vi "aal_Complex Modulator with Phase (complex input).vi"(7 "reset ?":bool, 8 "initial phase":dbl, 9 "fs":dbl=1024.0 min=-0.5 max=0.5 format="%.2f", 10 "frequency":dbl min=-0.5 max=0.5 format="%.2f", 11 "x":cdb[](array[numeric])) -> (3 "y":cdb[](array[numeric]))   [LabVIEW 2020, in "NI_AAL_SigProc.lvlib"]
doc: "Modulates the signal to frequency. The center frequency should be normalized (-0.5, 0.5)."
uses:
  <vilib>/Analysis/NI_AAL_SigProc.lvlib
  <resource>/lvanlys.dll
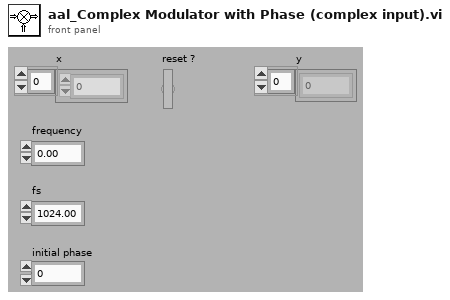
[diagram p1: front panel]
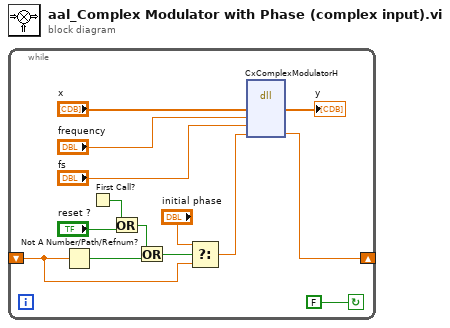
[diagram p0: block diagram]
diagram:
  n1 = while {
    shift-left: _ -> [w14]
    shift-right: [w9] -> _
    stop <- FALSE continue-if-true
    n2 = Not A Number/Path/Refnum?(number/path/refnum=w14) -> (NaN/Path/Refnum?=w5:bool)
    n3 = First Call?() -> (First Call?: T/F=w3:bool)
    n4 = Or(x=w3, y="reset ?") -> (x .or. y?=w1:bool)
    n5 = Or(x=w1, y=w5) -> (x .or. y?=w8:bool)
    n6 = Select(t="initial phase", s=w8, f=w14) -> (s? t:f=w10:dbl)
    n7 = dll-call lib="e:/builds/penguin/labview/branches/2020/dev/dist/resource/lvanlys.*" fn="CxComplexModulatorH"("x"="x", "fc"="frequency", "fs"="fs", "initial_phase"=w10) -> ("x"=→"y":cdb[], "initial_phase"=w9:dbl)  [unwired: 6 in, 2 out]
  }
